vi "Sequence step information.vi"() -> ()   [LabVIEW 2011]
uses:
  Sequence steps config..ctl
  Single criteria cluster.ctl
  Criteria types.ctl
  Boolean operation.ctl
panel:
  in  "Cluster":cluster{"Boolean":bool, "C1 op C2":T1}
  in  "Criteria 3":T2
  in  "Criteria 2":T2
  in  "C1 op C2":T1
  in  "Action":u16(ring)
  in  "Sequence step config":T4
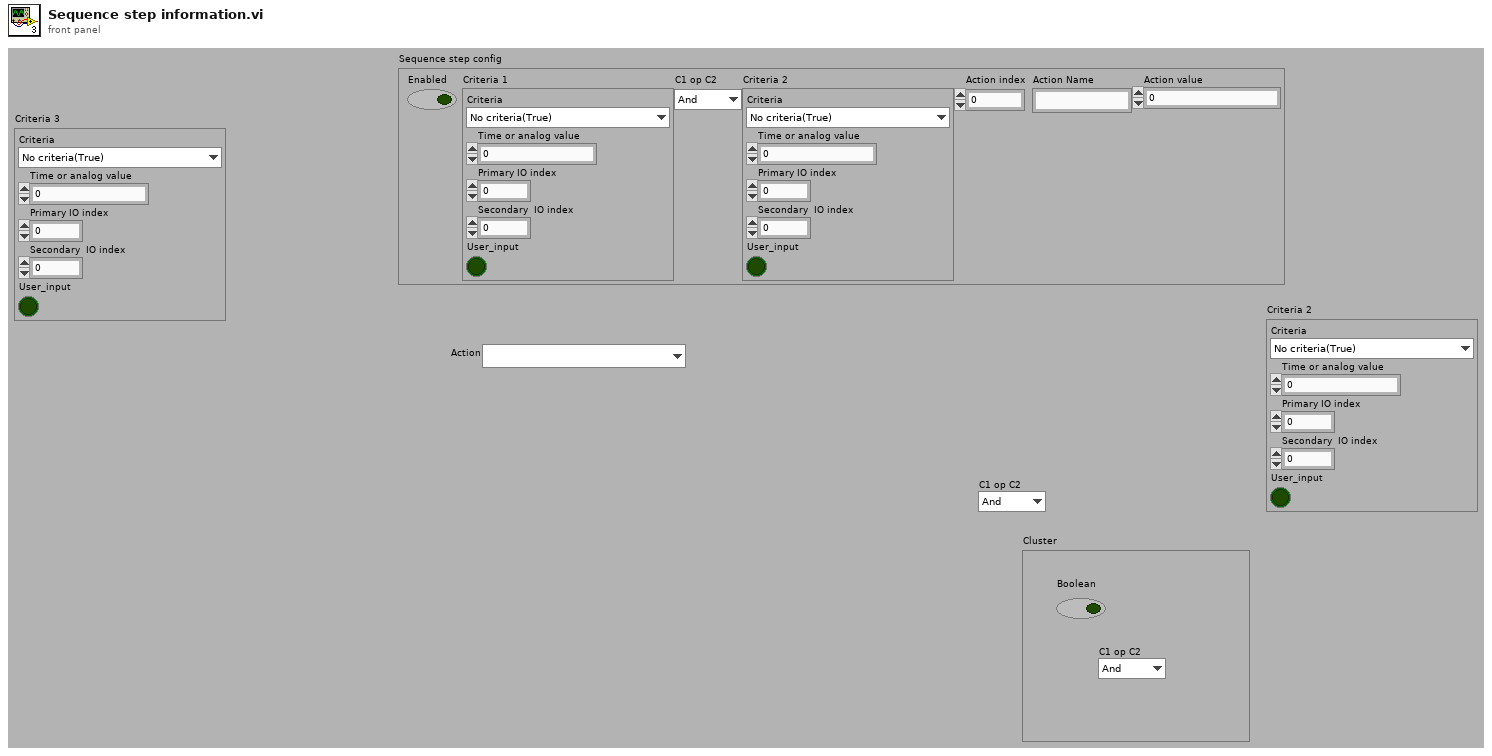
[diagram p1: front panel]
types:
  T1 = typedef "Boolean operation.ctl" = enum16{"And", "Or", "Xor", "Nand", "Nor", "Nxor", "Implies"}
  T2 = typedef "Single criteria cluster.ctl" = cluster{"Criteria":T3, "Time or analog value":dbl, "Primary IO index":i32, "Secondary  IO index":i32, "User_input":bool}
  T3 = typedef "Criteria types.ctl" = enum16{"No criteria(True)", "Time(s)", "Analog IO over", "Analog IO over or equal", "Analog IO under", "Analog IO under or equal", "Analog IO 1 minus Analog IO 2 over", "Digital IO True", "Digital IO False", "Operator approval"}
  T4 = typedef "Sequence steps config..ctl" = cluster{"Enabled":bool, "Criteria 1":T2, "C1 op C2":T1, "Criteria 2":T2, "Action index":i32, "Action Name":string, "Action value":dbl}
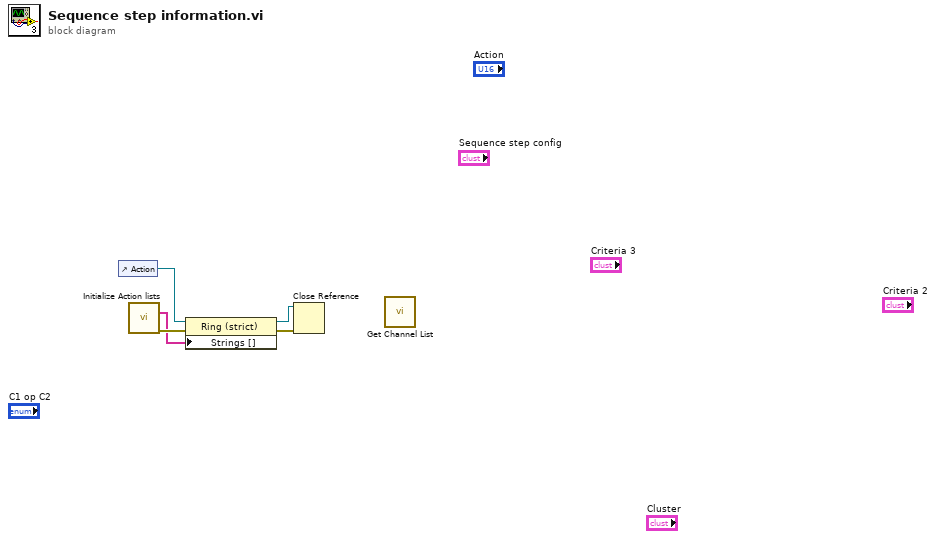
[diagram p0: block diagram]
diagram:
  n1 = control-ref of="Action"() -> (w5:refnum<vi>)
  n2 = call "Initialize Action lists.vi"() -> ("Action names"=w3:string[], "error out"=w4:errorcluster)  [unwired: 13 in, 1 out]
  n3 = property class="Ring (strict)"(reference=w5, error in=w4, "Strings []"=w3) -> (reference out=w1:refnum<vi>, error out=w2:errorcluster)
  n4 = Close Reference(reference=w1, error in (no error)=w2) -> ()  [unwired: 1 out]
  n5 = call "Get Channel List.vi"() -> ()  [unwired: 11 in, 5 out]
